vi "USB2CAN_Test.vi"() -> ()   [LabVIEW 2010]
panel:
  out "pCanGetMsg OUT":T1(array[cluster])
  in  "pCanGetMsg":T2
  in  "pCanSendMsg":T2={"ID"=1, "TimeStamp"=0, "RemoteFlag"=0, "ExternFlag"=0, "DataLen"=8, "Data[0]"=11, "Data[1]"=0, "Data[2]"=0, "Data[3]"=0, "Data[4]"=0, "Data[5]"=0, "Data[6]"=0, "Data[7]"=88, "__Res"=0}
  out "Get Msg Num":i32
  out "Success Sended Msg Num":i32
  in  "stop":bool
  in  "pCanConfig":T3={"CAN_BRP"=4, "CAN_SJW"=1, "CAN_BS1"=16, "CAN_BS2"=4, "CAN_Mode"=1, "CAN_ABOM"=1, "CAN_NART"=0, "CAN_RFLM"=0, "CAN_TXFP"=1}
  in  "CAN Channel":u8(ring) items=["CAN1", "CAN2"]
  in  "Device Index":i32(ring) items=["0", "1", "2", "3", "4", "5"]
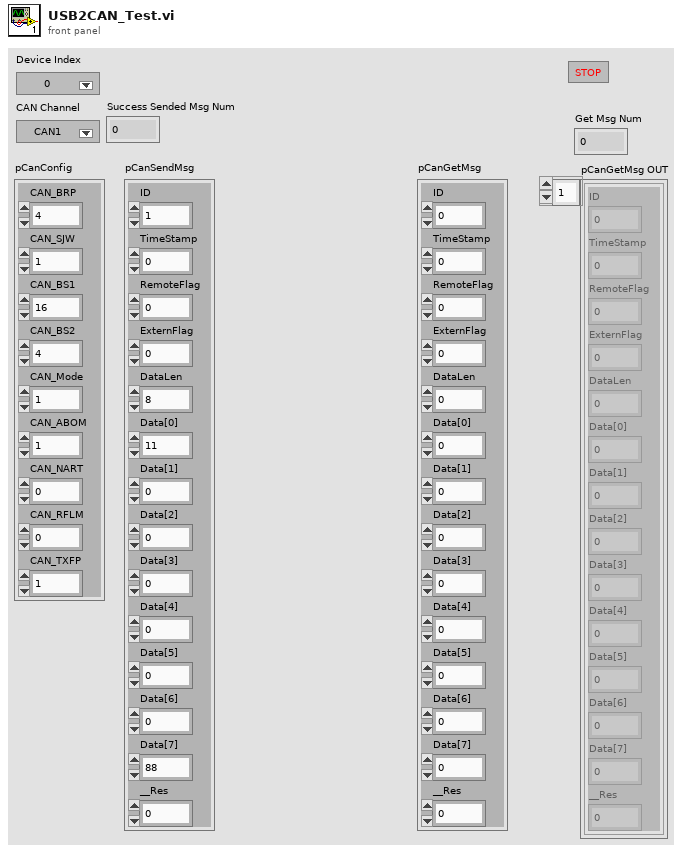
[diagram p1: front panel]
types:
  T1 = cluster{"ID":u32, "TimeStamp":u32, "RemoteFlag":u8, "ExternFlag":u8, "DataLen":u8, "Data[0]":u8, "Data[1]":u8, "Data[2]":u8, "Data[3]":u8, "Data[4]":u8, "Data[5]":u8, "Data[6]":u8, "Data[7]":u8, "__Res":u8}[]
  T2 = cluster{"ID":u32, "TimeStamp":u32, "RemoteFlag":u8, "ExternFlag":u8, "DataLen":u8, "Data[0]":u8, "Data[1]":u8, "Data[2]":u8, "Data[3]":u8, "Data[4]":u8, "Data[5]":u8, "Data[6]":u8, "Data[7]":u8, "__Res":u8}
  T3 = cluster{"CAN_BRP":u32, "CAN_SJW":u8, "CAN_BS1":u8, "CAN_BS2":u8, "CAN_Mode":u8, "CAN_ABOM":u8, "CAN_NART":u8, "CAN_RFLM":u8, "CAN_TXFP":u8}
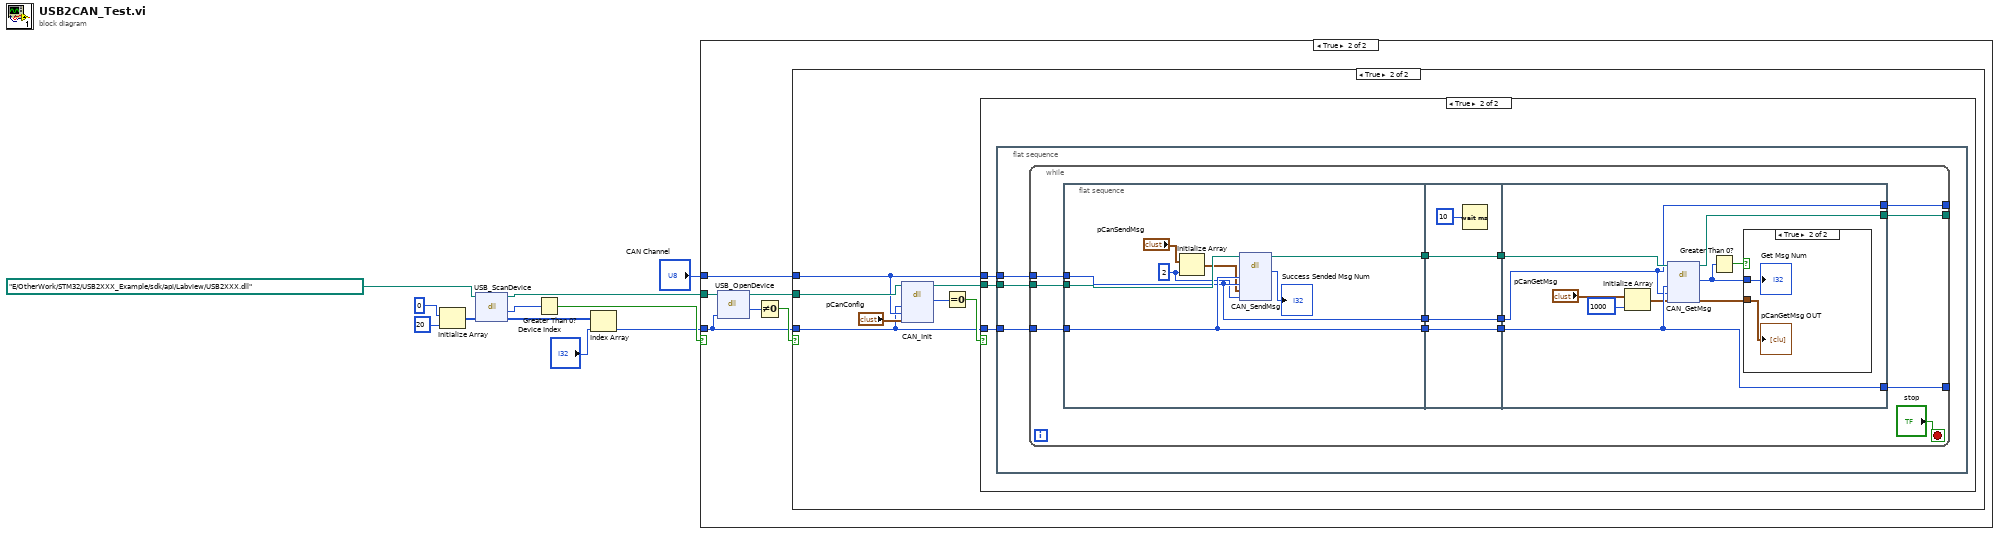
[diagram p0: block diagram]
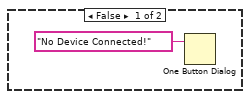
[diagram p2: hidden frame]
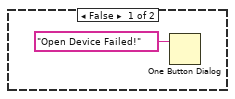
[diagram p3: hidden frame]
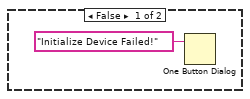
[diagram p4: hidden frame]
diagram:
  n1 = Initialize Array(0, 20 ("dimension size")) -> (w11:i32[])
  n2 = dll-call lib="E:/OtherWork/STM32/USB2XXX_Example/sdk/api/Labview/USB2XXX.dll" fn="USB_ScanDevice"(path in=path "E:/OtherWork/STM32/USB2XXX_Example/sdk/api/Labview/USB2XXX.dll", "pDevNum"=w11) -> (path out=w2:path, "return type"=w7:i32, "pDevNum"=w8:i32[])  [unwired: 2 in, 1 out]
  n3 = Greater Than 0?(x=w7) -> (x > 0?=w6:bool)
  n4 = Index Array(array=w8, index="Device Index") -> (element=w4:i32)
  n5 = case shown="True" w6 {
    tunnel: w4 -> [_ w15]
    tunnel: w2 -> [_ w16]
    tunnel: "CAN Channel" -> [_ w14]
    frame False {
      n6 = One Button Dialog(message="No Device Connected!") -> ()  [unwired: 1 in, 1 out]
    }
    frame True {
      n7 = dll-call lib="E:/OtherWork/STM32/USB2XXX_Example/sdk/api/Labview/USB2XXX.*" fn="USB_OpenDevice"(path in=w16, "DevHandle"=w15) -> (path out=w13:path, "return type"=w18:u8)  [unwired: 3 in, 1 out]
      n8 = Not Equal To 0?(x=w18) -> (x != 0?=w17:bool)
      n9 = case shown="True" w17 {
        tunnel: w13 -> [_ w25]
        tunnel: w15 -> [_ w22]
        tunnel: w14 -> [_ w24]
        frame False {
          n10 = One Button Dialog(message="Open Device Failed!") -> ()  [unwired: 1 in, 1 out]
        }
        frame True {
          n11 = dll-call lib="E:/OtherWork/STM32/USB2XXX_Example/sdk/api/Labview/USB2XXX.*" fn="CAN_Init"(path in=w25, "DevHandle"=w22, "CANIndex"=w24, "pCanConfig"="pCanConfig") -> (path out=w20:path, "return type"=w21:i32)  [unwired: 5 in, 1 out]
          n12 = Equal To 0?(x=w21) -> (x = 0?=w26:bool)
          n13 = case shown="True" w26 {
            tunnel: w20 -> [_ w28]
            tunnel: w22 -> [_ w29]
            tunnel: w24 -> [_ w30]
            frame False {
              n14 = One Button Dialog(message="Initialize Device Failed!") -> ()  [unwired: 1 in, 1 out]
            }
            frame True {
              n15 = flat-sequence {
                tunnel: w28 -> [w33]
                tunnel: w30 -> [w32]
                tunnel: w29 -> [w31]
                frame #0 {
                  n16 = while {
                    tunnel: w33 -> [w46]
                    tunnel: w32 -> [w45]
                    tunnel: w31 -> [w44]
                    tunnel: [w36] -> _
                    tunnel: [w35] -> _
                    tunnel: [w34] -> _
                    stop <- "stop" stop-if-true
                    n17 = flat-sequence {
                      tunnel: w46 -> [w54]
                      tunnel: w45 -> [w52]
                      tunnel: w44 -> [w53]
                      tunnel: [w52] -> w42
                      tunnel: [w53] -> w40
                      tunnel: [w48] -> w38
                      tunnel: w42 -> [w57]
                      tunnel: [w57] -> w41
                      tunnel: w40 -> [w56]
                      tunnel: [w56] -> w39
                      tunnel: w38 -> [w55]
                      tunnel: [w55] -> w37
                      tunnel: w41 -> [w65]
                      tunnel: w39 -> [w66]
                      tunnel: w37 -> [w67]
                      tunnel: [w63] -> w36
                      tunnel: [w66] -> w35
                      tunnel: [w65] -> w34
                      frame #0 {
                        w50 = u32 2 ("dimension size")
                        n18 = Initialize Array("pCanSendMsg", w50) -> (w51:T1)
                        n19 = dll-call lib="E:/OtherWork/STM32/USB2XXX_Example/sdk/api/Labview/USB2XXX.*" fn="CAN_SendMsg"(path in=w54, "DevHandle"=w53, "CANIndex"=w52, "pCanSendMsg"=w51, "SendMsgNum"=w50) -> (path out=w48:path, "return type"=→"Success Sended Msg Num":i32)  [unwired: 6 in, 1 out]
                      }
                      frame #1 {
                        n20 = Wait (ms)(milliseconds to wait=u32 10 ("等待时间（毫秒）")) -> ()  [unwired: 1 out]
                      }
                      frame #2 {
                        n21 = Initialize Array("pCanGetMsg", 1000 ("BufferSize")) -> (w64:T1)
                        n22 = dll-call lib="E:/OtherWork/STM32/USB2XXX_Example/sdk/api/Labview/USB2XXX.*" fn="CAN_GetMsg"(path in=w67, "DevHandle"=w66, "CANIndex"=w65, "pCanGetMsg"=w64) -> (path out=w63:path, "return type"=w60:i32, "pCanGetMsg"=w61:T1)  [unwired: 4 in, 1 out]
                        n23 = Greater Than 0?(x=w60) -> (x > 0?=w59:bool)
                        n24 = case shown="True" w59 {
                          tunnel: w60 -> [_ w70]
                          tunnel: w61 -> [_ w69]
                          frame False {
                          }
                          frame True {
                            "Get Msg Num" <- w70
                            "pCanGetMsg OUT" <- w69
                          }
                        }
                      }
                    }
                  }
                }
              }
            }
          }
        }
      }
    }
  }
